vi "Read Property.vi"(6 "Initialized in":bool, 8 "error in (no error)":errorcluster, 9 "Programming Mode In":T2[](array[typedef]), 10 "References":refnum<vi>[](array[refnum]), 11 "Refnum in":refnum<k20>) -> (0 "error out":errorcluster, 1 "Programming Mode Out":T2[](array[typedef]), 2 "Slot":i32, 3 "Refnum out":refnum<k20>, 4 "Initialized Out":bool)   [LabVIEW 2019, in "SEECD System Explorer.lvlib"]
doc: "Get values available (taking into account Model), Read current property value for populated slots, set respective Control."
uses:
  SEECD System Explorer.lvlib
  Includes/Modules.lvlibp/RSI Module/Module Models.ctl
  Type Defs/Slot Programming Mode.ctl
  Type Defs/Slot - Configuration.ctl
  <resource>/objmgr/nicriosae.rc
  Includes/Modules.lvlibp/RSI Module/RSI Module.lvclass
panel:
  in  "Module Name":string
  in  "Slot":T1={"Slot"="", "Module Name"="", "Current Prog Mode"="", "New Prog Mode"=enum."Scan Engine"}
  in  "Module":T3
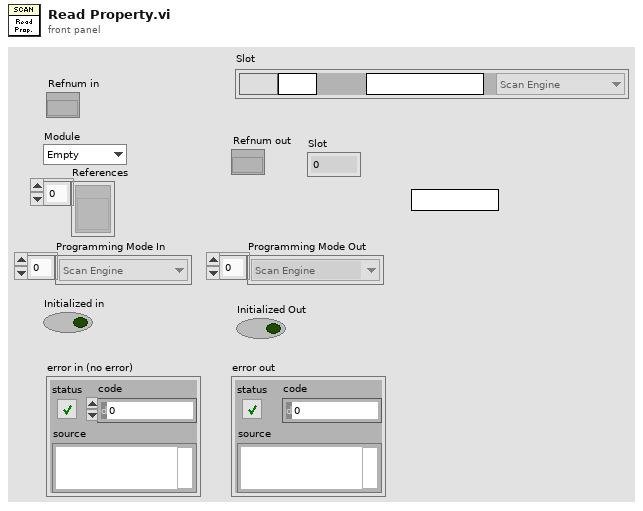
[diagram p1: front panel]
types:
  T1 = typedef "SEECD System Explorer.lvlib/Slot - Configuration.ctl" = cluster{"Slot":string, "Module Name":string, "Current Prog Mode":string, "New Prog Mode":T2}
  T2 = typedef "SEECD System Explorer.lvlib/Slot Programming Mode.ctl" = enum16{"Don't Modify", "Scan Engine", "LabVIEW FPGA", "NI-DAQmx"}
  T3 = typedef "Modules.lvlibp/RSI Module.lvclass/Module Models.ctl" = enum16{"Empty", "NI 9201", "NI 9203", "NI 9205", "NI 9206", "NI 9207", "NI 9208", "NI 9209", "NI 9210", "NI 9211", "NI 9212", "NI 9213", "NI 9214", "NI 9215", "NI 9216", "NI 9217", "NI 9219", "NI 9220", "NI 9221", "NI 9222", "NI 9223", "NI 9224", "NI 9225", "NI 9226", "NI 9227", "NI 9228", "NI 9229", "NI 9233", "NI 9234", "NI 9235", "NI 9236", "NI 9237", "NI 9239", "NI 9242", "NI 9244", "NI 9253", "NI 9263", "NI 9264", "NI 9265", "NI 9266", "NI 9269", "NI 9344", "NI 9350", "NI 9375", "NI 9401", "NI 9402", "NI 9403", "NI 9411", "NI 9421", "NI 9422", "NI 9423", "NI 9425", "NI 9426", "NI 9435", "NI 9436", "NI 9437", "NI 9472", "NI 9474", "NI 9475", "NI 9476", "NI 9477", "NI 9478", "NI 9481", "NI 9482", "NI 9485"}
  T4 = enum8{"Enabled", "Disabled", "Disabled and Grayed Out"}
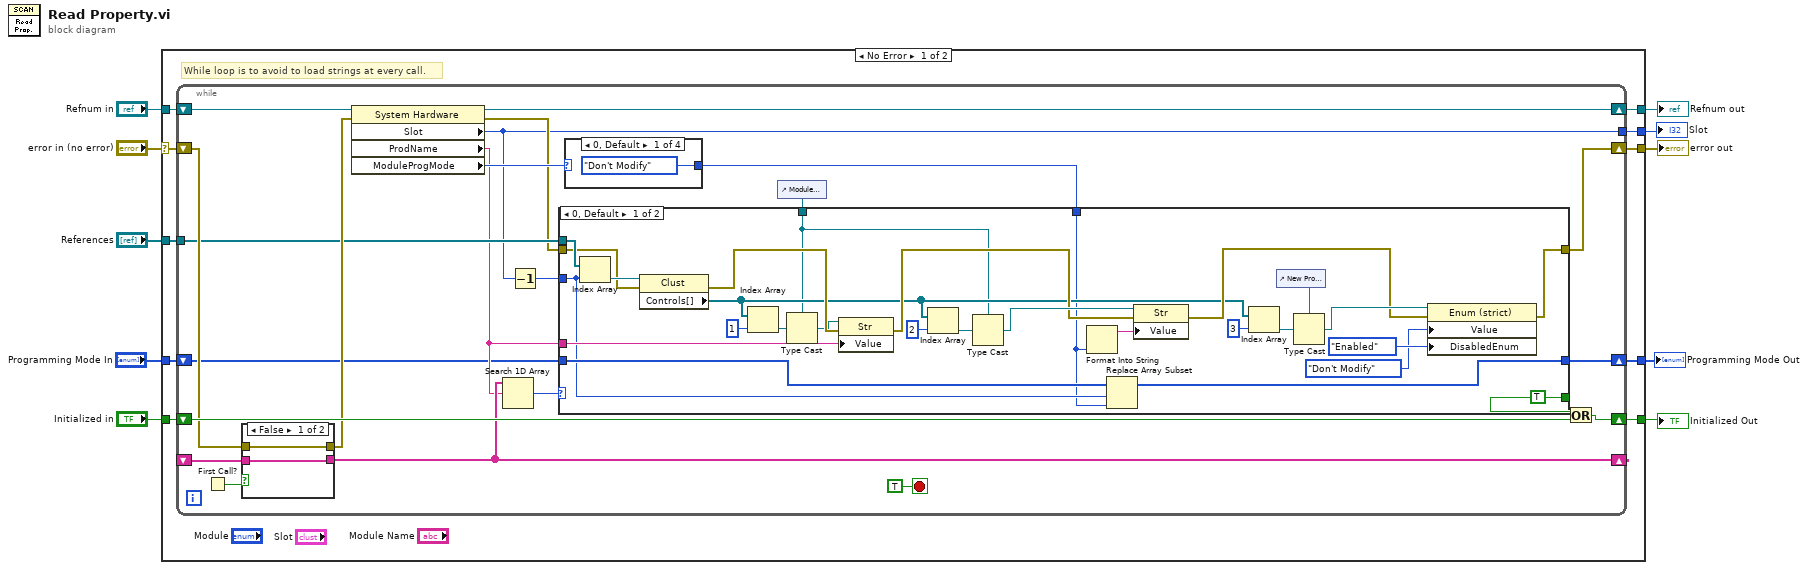
[diagram p0: block diagram]
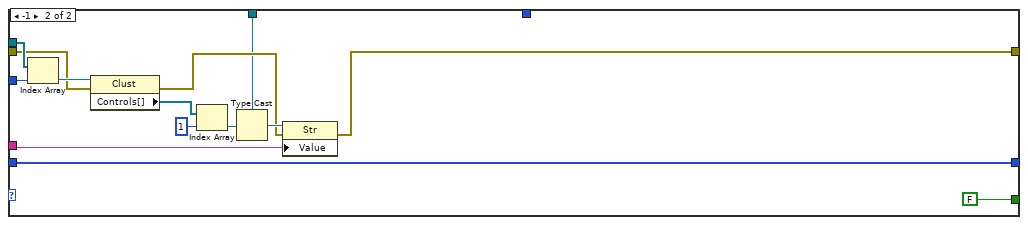
[diagram p2: hidden frame]
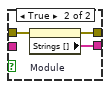
[diagram p3: hidden frame]
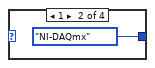
[diagram p4: hidden frame]
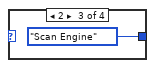
[diagram p5: hidden frame]
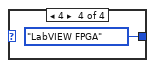
[diagram p6: hidden frame]
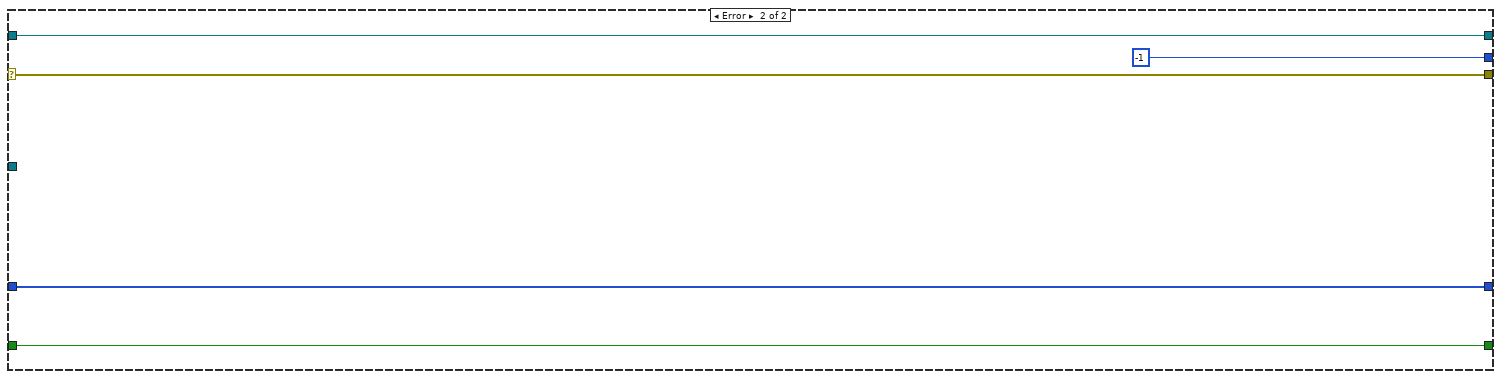
[diagram p7: hidden frame]
diagram:
  n1 = case shown="No Error" "error in (no error)" {
    selector: "error in (no error)" -> [w15 w98]
    tunnel: [w20 w97] -> w10
    tunnel: "Initialized in" -> [w19 w97]
    tunnel: [w18 w98] -> w8
    tunnel: [w17 w99] -> w7
    tunnel: "Refnum in" -> [w16 w99]
    tunnel: "References" -> [w14 _]
    tunnel: "Programming Mode In" -> [w13 w96]
    tunnel: [w12 w96] -> w3
    tunnel: [w11 -1 ("Slot")] -> w2
    frame No Error {
      # "While loop is to avoid to load strings at every call."
      n2 = while {
        shift-right: [w43] -> w20
        shift-left: w19 -> [w42]
        shift-right: [w40] -> w17
        shift-left: w16 -> [w39]
        shift-right: [w32] -> w18
        shift-left: w15 -> [w34]
        shift-right: [w33] -> _
        shift-left: _ -> [w35]
        tunnel: w14 -> [w30]
        shift-right: [w25] -> w12
        shift-left: w13 -> [w26]
        tunnel: [w21] -> w11
        stop <- TRUE stop-if-true
        n3 = First Call?() -> (First Call?: T/F=w37:bool)
        n4 = case shown="False" w37 {
          tunnel: [w87 w90] -> w36
          tunnel: [w86 w89] -> w33
          tunnel: w35 -> [w86 _]
          tunnel: w34 -> [w87 w88]
          frame False {
          }
          frame True {
            n5 = property on="Module" class="Enum (strict)"(error in=w88) -> (error out=w90:errorcluster, "Strings []"=w89:string[])  [unwired: 1 in, 1 out]
          }
        }
        n6 = property class="System Hardware"(reference=w39, error in=w36) -> (reference out=w40:refnum<k20>, error out=w28:errorcluster, "Slot"=w21:i32, "ProdName"=w27:string, "ModuleProgMode"=w29:u32)
        n7 = Search 1D Array(1D array=w33, element=w27) -> (index of element=w31:i32)  [unwired: 1 in]
        n8 = Decrement(x=w21) -> (x-1=w22:i32)
        n9 = case shown="0, Default" w29 {
          tunnel: [Slot_Programming_Mode."Don't Modify" ("Value") Slot_Programming_Mode."NI-DAQmx" ("Value") Slot_Programming_Mode."Scan Engine" ("Value") Slot_Programming_Mode."LabVIEW FPGA" ("Value")] -> w23
          frame 0, Default {
          }
          frame 1 {
          }
          frame 2 {
          }
          frame 4 {
          }
        }
        n10 = control-ref of="Module Name"() -> (w24:refnum<vi>)
        n11 = case shown="0, Default" w31 {
          tunnel: [TRUE FALSE] -> w41
          tunnel: w28 -> [w64 w80]
          tunnel: [w48 w75] -> w32
          tunnel: w30 -> [w65 w83]
          tunnel: w22 -> [w57 w82]
          tunnel: w27 -> [w63 w74]
          tunnel: w26 -> [w58 w84]
          tunnel: [w56 w84] -> w25
          tunnel: w24 -> [w44 w72]
          tunnel: w23 -> [w46 _]
          frame 0, Default {
            n12 = Index Array(array=w65, index=w57) -> (element=w67:refnum<vi>)
            n13 = property class="Clust"(reference=w67, error in=w64) -> (error out=w70:errorcluster, "Controls[]"=w50:refnum<vi>[])  [unwired: 1 out]
            n14 = Index Array(array=w50, index=1) -> (element=w68:refnum<vi>)
            n15 = Type Cast(type=w44, x=w68) -> (*(type *) &x=w69:refnum<vi>)
            n16 = property class="Str"(reference=w69, error in=w70, "Value"=w63) -> (error out=w59:errorcluster)  [unwired: 1 out]
            n17 = Index Array(array=w50, index=2) -> (element=w61:refnum<vi>)
            n18 = Type Cast(type=w44, x=w61) -> (*(type *) &x=w60:refnum<vi>)
            n19 = Format Into String(w46) -> (resulting string=w45:string)  [unwired: 3 in, 1 out]
            n20 = Replace Array Subset(array=w58, new element=w46, index=w57) -> (w56:T2[])
            n21 = property class="Str"(reference=w60, error in=w59, "Value"=w45) -> (error out=w51:errorcluster)  [unwired: 1 out]
            n22 = Index Array(array=w50, index=3) -> (element=w53:refnum<vi>)
            n23 = control-ref of="New Prog Mode"() -> (w54:refnum<vi>)
            n24 = Type Cast(type=w54, x=w53) -> (*(type *) &x=w55:refnum<vi>)
            n25 = property class="Enum (strict)"(reference=w55, error in=w51, "Value"=Slot_Programming_Mode."Don't Modify", "DisabledEnum"=T4."Enabled" ("Disabled")) -> (error out=w48:errorcluster)  [unwired: 1 out]
          }
          frame -1 {
            n26 = Index Array(array=w83, index=w82) -> (element=w81:refnum<vi>)
            n27 = property class="Clust"(reference=w81, error in=w80) -> (error out=w76:errorcluster, "Controls[]"=w73:refnum<vi>[])  [unwired: 1 out]
            n28 = Index Array(array=w73, index=1) -> (element=w78:refnum<vi>)
            n29 = Type Cast(type=w72, x=w78) -> (*(type *) &x=w77:refnum<vi>)
            n30 = property class="Str"(reference=w77, error in=w76, "Value"=w74) -> (error out=w75:errorcluster)  [unwired: 1 out]
          }
        }
        n31 = Or(x=w41, y=w42) -> (x .or. y?=w43:bool)
      }
    }
    frame Error {
    }
  }
  "Initialized Out" <- w10
  "error out" <- w8
  "Refnum out" <- w7
  "Programming Mode Out" <- w3
  "Slot" <- w2
